vi "ZADD.vi"(0 "TCP session out":refnum<k5>, 1 "Key":string, 5 "Scores":string[](array[string]), 7 "Members":string[](array[string]), 11 "error in":errorcluster) -> (4 "TCP session out":refnum<k5>, 6 "Data":T1, 15 "error out":errorcluster)   [LabVIEW 2023]
uses:
  SubVIs/Controls/redis-data.ctl
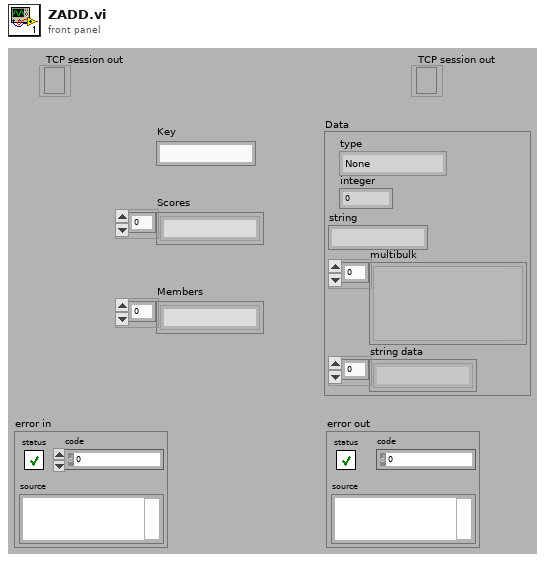
[diagram p1: front panel]
types:
  T1 = typedef "redis-data.ctl" = cluster{"type":enum16{"None", "Error", "Status", "Nil", "Integer", "String", "Multibulk"}, "integer":i64, "string":string, "multibulk":variant[], "string data":string[]}
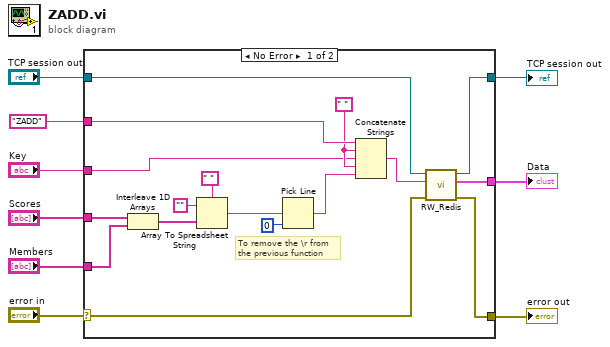
[diagram p0: block diagram]
diagram:
  n1 = case shown="No Error" "error in" {
    selector: "error in" -> [w20 w28]
    tunnel: "Scores" -> [w15 _]
    tunnel: "ZADD" -> [w13 _]
    tunnel: "TCP session out" -> [w17 w27]
    tunnel: [w19 w28] -> w5
    tunnel: [w18 _] -> w4
    tunnel: [w10 w27] -> w3
    tunnel: "Members" -> [w16 _]
    tunnel: "Key" -> [w11 _]
    frame No Error {
      w12 = " "
      # "To remove the \\r from\nthe previous function"
      n2 = Interleave 1D Arrays(w15, w16) -> (w14:string[])
      n3 = Array To Spreadsheet String(delimiter (Tab)=" ", array=w14, 3:"" ("format string")) -> (spreadsheet string=w23:string)
      n4 = Pick Line(multi-line string=w23, line index=0) -> (output string=w24:string)  [unwired: 1 in]
      n5 = Concatenate Strings(w13, w12, w11, w12, w24) -> (w21:string)
      n6 = call "RW_Redis.vi"("error in"=w20, "command"=w21, "TCP session in"=w17) -> ("error out"=w19:errorcluster, "Data"=w18:T1, "TCP session out"=w10:refnum<k5>)  [unwired: 6 in]
    }
    frame Error {
    }
  }
  "error out" <- w5
  "Data" <- w4
  "TCP session out" <- w3
